vi "_ConnectorPaneEditor_Inicjalize.vi"(8 "error in (no error)":errorcluster, 11 "ConnectorPaneEditor in":refnum<class "_ConnectorPaneEditor.lvclass">) -> (0 "error out":errorcluster, 3 "ConnectorPaneEditor out":refnum<class "_ConnectorPaneEditor.lvclass">)   [LabVIEW 2014, in "_ConnectorPaneEditor.lvclass"]
uses:
  _ConnectorPaneEditor.lvclass
  _ConnectorPaneEditor.lvclass/_ConnectorPaneEditor.ctl
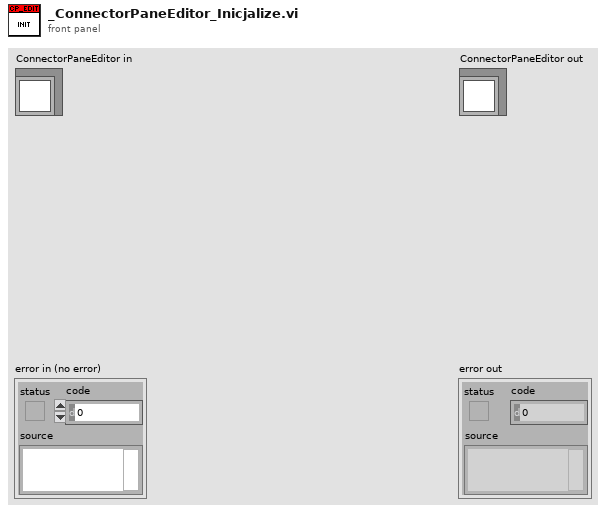
[diagram p1: front panel]
types:
  T1 = enum16{"Invalid Wire Rule", "Required", "Recommended", "Optional", "Dynamic Dispatch"}[]
  T2 = typedef "LVRectTypeDef.ctl" = cluster{"Left":i16, "Top":i16, "Right":i16, "Bottom":i16}
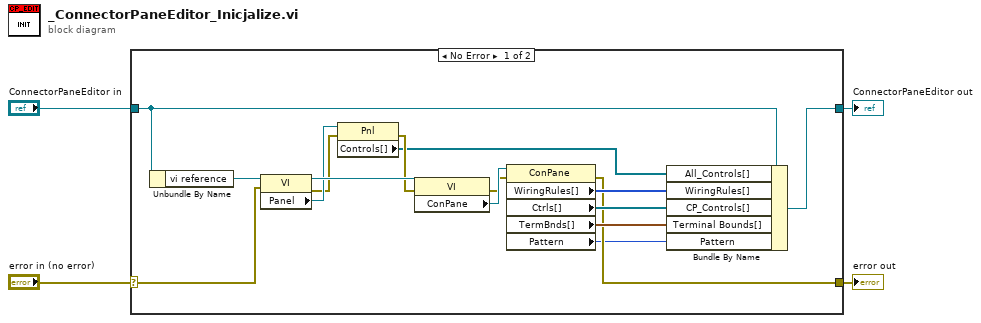
[diagram p0: block diagram]
diagram:
  n1 = case shown="No Error" "error in (no error)" {
    selector: "error in (no error)" -> [w7 w22]
    tunnel: [w6 w22] -> w3
    tunnel: [w9 w21] -> w1
    tunnel: "ConnectorPaneEditor in" -> [w10 w21]
    frame No Error {
      n2 = Unbundle By Name(w10) -> ("vi reference"=w17:refnum<vi>)
      n3 = property class="VI"(reference=w17, error in=w7) -> (reference out=w16:refnum<vi>, error out=w14:errorcluster, "Panel"=w15:refnum<vi>)
      n4 = property class="Pnl"(reference=w15, error in=w14) -> (error out=w13:errorcluster, "Controls[]"=w12:refnum<vi>[])  [unwired: 1 out]
      n5 = property class="VI"(reference=w16, error in=w13) -> (error out=w19:errorcluster, "ConPane"=w20:refnum<vi>)  [unwired: 1 out]
      n6 = property class="ConPane"(reference=w20, error in=w19) -> (error out=w6:errorcluster, "WiringRules[]"=w11:T1, "Ctrls[]"=w18:refnum<vi>[], "TermBnds[]"=w8:T2[], "Pattern"=w5:u32)  [unwired: 1 out]
      n7 = Bundle By Name(cluster=w10, "All_Controls[]"=w12, "WiringRules[]"=w11, "CP_Controls[]"=w18, "Terminal Bounds[]"=w8, "Pattern"=w5) -> (w9:refnum<class "_ConnectorPaneEditor.lvclass">)
    }
    frame Error {
    }
  }
  "error out" <- w3
  "ConnectorPaneEditor out" <- w1
